vi "Check LDA Data Rate.vi"   [LabVIEW 2020]
uses:
  Globals/Meas_global.vi
  Globals/LDA_global.vi
  Globals/Preference_global.vi
types:
  T1 = typedef "Analysis_info_cluster.ctl" = cluster{"Colour":u32, "Inst type":T2, "Inst name":string, "Symbol":string, "Code name":string, "Extra Info":string, "Inst Array":T3, "Extra Titles":string[], "Extra Values":string[], "U":dbl, "u^2":dbl, "u^3":dbl, "u^4":dbl, "Skew_u":dbl, "Kurt_u":dbl, "Sd Error in Mean":dbl, "% u'/U":dbl, "X":dbl, "Y":dbl, "Z":dbl, "Timescale integral Estimate":dbl, "Sd Error in Variance":dbl, "Calib File":path, "Calib Constants":dbl[], "Output Position":bool, "Stats":enum16{"None", "Basic", "Full"}, "Av Sampling Rate":dbl, "Av No of Samples":dbl, "Total Meas Time (s)":dbl, "ADAM Ch Name":string, "Max value":dbl, "Min value":dbl, "Req Sample Rate Hz":dbl, "Sync Delay Time (s)":dbl, "Ch No":i16, "Device":string, "Use Latest Calib":bool, "Port":string, "Metadata Ch Names":string[], "Metadata Ch Values":string[], "Label":string}
  T2 = typedef "Inst_type.ctl" = enum16{"Raw voltage", "Raw with zero offsetting", "Propeller anemometer", "Pressure Transducer", "Pitot-static tube", "Hot wire", "Cross wire 1", "Cross wire 2", "Generic Linear", "Generic Polynomial", "Generic BackPoly", "Fast FID", "Thermocouple", "Cold wire", "Pulsed Wire", "LDA Vel", "LDA Tran time", "LDA Arr time", "Microphone"}
  T3 = typedef "Instrument_Array.ctl" = enum16{"PWA", "LDA", "Analogue"}
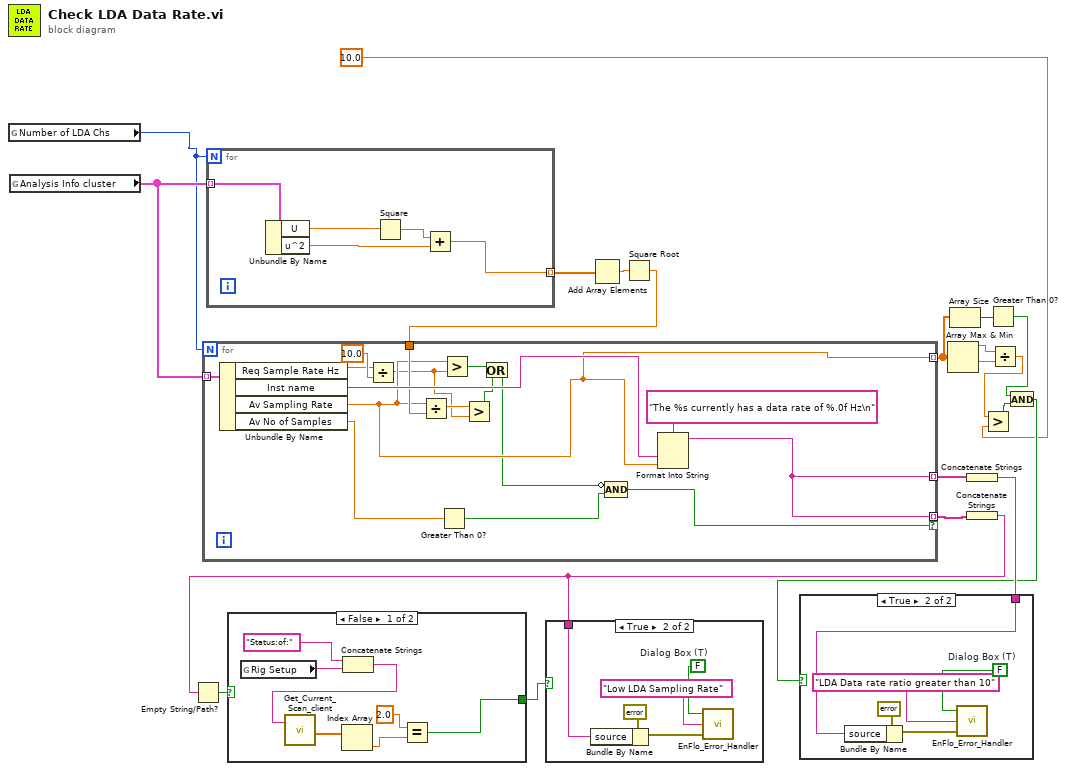
[diagram p0: block diagram]
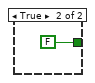
[diagram p4: hidden frame]
diagram:
  n1 = global read "LDA_global.vi" "Number of LDA Chs"() -> (w1:i32)
  n2 = global read "Meas_global.vi" "Analysis Info cluster"() -> (w4:T1[])
  n3 = for {
    N: w1 -> [_]
    tunnel: w4 -> [w25] mode=indexing
    tunnel: [w21] -> w6 mode=indexing
    n4 = Unbundle By Name(w25) -> ("U"=w24:dbl, "u^2"=w22:dbl)
    n5 = Square(x=w24) -> (x^2=w23:dbl)
    n6 = Add(x=w23, y=w22) -> (x+y=w21:dbl)
  }
  n7 = Add Array Elements(numeric array=w6) -> (sum=w5:dbl)
  n8 = Square Root(x=w5) -> (sqrt(x)=w3:dbl)
  n9 = for {
    N: w1 -> [_]
    tunnel: w4 -> [w41] mode=indexing
    tunnel: [w32] -> w9 mode=indexing
    tunnel: [w30] -> w17 mode=indexing if=w27
    tunnel: [w30] -> w19 mode=indexing
    tunnel: w3 -> [w38]
    n10 = Unbundle By Name(w41) -> ("Req Sample Rate Hz"=w35:dbl, "Inst name"=w40:string, "Av Sampling Rate"=w32:dbl, "Av No of Samples"=w28:dbl)
    n11 = Divide(x=w35, y=10.0) -> (x/y=w29:dbl)
    n12 = Divide(x=w32, y=w38) -> (x/y=w36:dbl)
    n13 = Greater Than 0?(x=w28) -> (x > 0?=w26:bool)
    n14 = Greater?(x=w32, y=w29) -> (0:w33:bool)
    n15 = Greater?(x=w36, y=w29) -> (0:w34:bool)
    n16 = Or(x=w33, y=w34) -> (x .or. y?=w31:bool)
    n17 = Compound Arithmetic op=AND(invert w31, w26) -> (w27:bool)
    n18 = Format Into String(format string="The %s currently has a data rate of %.0f Hz\n", w40, w32) -> (resulting string=w30:string)  [unwired: 2 in, 1 out]
  }
  n19 = Array Max & Min(array=w9) -> (max value=w11:dbl, min value=w12:dbl)  [unwired: 2 out]
  n20 = Array Size(array=w9) -> (size(s)=w10:i32)
  n21 = Concatenate Strings(w19) -> (w20:string)
  n22 = Concatenate Strings(w17) -> (w18:string)
  n23 = Empty String/Path?(string/path=w18) -> (empty?=w7:bool)
  n24 = case shown="False" w7 {
    tunnel: [w43 FALSE] -> w8
    frame False {
      n25 = global read "Preference_global.vi" "Rig Setup"() -> (w47:string)
      n26 = Concatenate Strings("Status:of:", w47) -> (w42:string)
      n27 = call "Get_Current_Scan_client.vi"("singleChannel"=w42) -> ("Numerical Values"=w46:dbl[])  [unwired: 1 in, 3 out]
      n28 = Index Array(array=w46) -> (element=w45:dbl)  [unwired: 1 in]
      n29 = Equal?(x=2.0, y=w45) -> (x = y?=w43:bool)
    }
    frame True {
    }
  }
  n30 = case shown="True" w8 {
    tunnel: w18 -> [_ w50]
    frame False {
    }
    frame True {
      w53 = FALSE  # Dialog Box (T)
      n31 = Bundle By Name(cluster=errorcluster {"status"=TRUE, "code"=0, "source"=""} ("error in (no error)"), "source"=w50) -> (w52:errorcluster)
      n32 = call "EnFlo_Error_Handler.vi"("error in (no error)"=w52, "Error Type"="Low LDA Sampling Rate", "Dialog Box (F)"=w53) -> ()  [unwired: 3 out]
    }
  }
  n33 = Greater Than 0?(x=w10) -> (x > 0?=w14:bool)
  n34 = Divide(x=w11, y=w12) -> (x/y=w16:dbl)
  n35 = Greater?(x=w16, y=10.0 ("f")) -> (0:w13:bool)
  n36 = And(x=w14, y=w13) -> (x .and. y?=w15:bool)
  n37 = case shown="True" w15 {
    tunnel: w20 -> [_ w55]
    frame False {
    }
    frame True {
      w58 = FALSE  # Dialog Box (T)
      n38 = Bundle By Name(cluster=errorcluster {"status"=TRUE, "code"=0, "source"=""} ("error in (no error)"), "source"=w55) -> (w57:errorcluster)
      n39 = call "EnFlo_Error_Handler.vi"("error in (no error)"=w57, "Error Type"="LDA Data rate ratio greater than 10", "Dialog Box (F)"=w58) -> ()  [unwired: 3 out]
    }
  }
